vi "Periodic Tasks.vi"(8 "error in":errorcluster) -> ()   [LabVIEW 2020]
doc: "This VI runs in parallel to other tasks. It can contain as many user-defined periodic loops as you need. These can carry out PID or other sorts of timed response."
uses:
  <vilib>/Rock Robotics/WPI/ThirdParty/Phoenix-LabVIEW/Motor Controller/Controls/CTRE_Phoenix_MotorControl_ControlMode.ctl
  <vilib>/Analysis/coordinate.llb/Angle Range (Degree).ctl
  <vilib>/Analysis/coordinate.llb/Angle Units.ctl
  <vilib>/Analysis/coordinate.llb/Wrap Angle (scalar).vi
  globals.vi
  <vilib>/Rock Robotics/WPI/ThirdParty/Phoenix-LabVIEW/Pigeon IMU/CTRE_PigeonIMU_GetYPR.vi
  <vilib>/Rock Robotics/WPI/ThirdParty/Phoenix-LabVIEW/CANCoder/Get/CTRE_Phoenix_CANcoder_GetSensorData.vi
  <vilib>/Rock Robotics/WPI/ThirdParty/Phoenix-LabVIEW/CANCoder/Set/CTRE_Phoenix_CANcoder_SetPositionToAbsolute.vi
  <vilib>/Rock Robotics/WPI/ThirdParty/Phoenix-LabVIEW/Motor Controller/Get/CTRE_Phoenix_MotorController_GetSelectedSensorData.vi
  TitanLib/Lib/TitanLib.lvlib
  <vilib>/Analysis/NI_AAL_Angle.lvlib
panel:
  out "Pose Estimation (in) 3":cluster{"Pose[0]":dbl, "Pose[1]":dbl}[](graph)
  in  "wheel offset":dbl
  in  "Reset Odometry?":bool
  in  "Reset Encoders?":bool
  out "Encoders":dbl[](array[numeric])
  in  "Zero Pigeon?":bool
  out "Pose Estimation (in) 2":T1(graph)
  out "Pose Estimation (in)":cluster{"X":dbl, "Y":dbl}[](graph)
  in  "Drive Speed Multiplier":dbl=1.0
  in  "Enable Drive Motors?":bool=TRUE
  in  "Acceleration":i32=8192
  in  "Cruise Velocity":i32=20000
  in  "I":dbl
  in  "D":dbl=50.0
  in  "P":dbl=1.0
  in  "Set PIDF":bool
  out "Loop Time (ms)":u32(graph)
  # "Pos"
  # "Abs"
  # "Pos"
  # "Abs"
  # "Pos"
  # "Abs"
  # "Pos"
  # "Abs"
  # "30ft x 30ft"
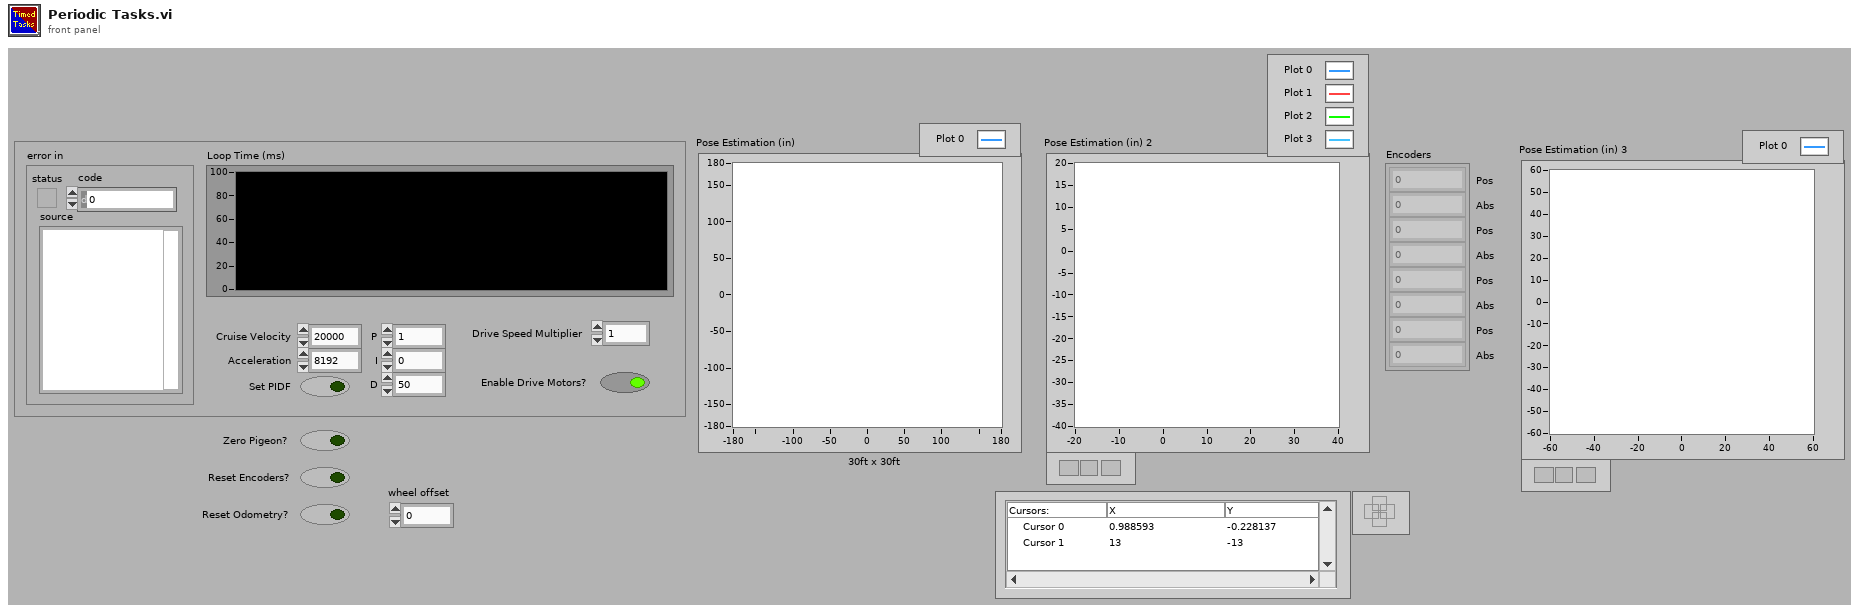
[diagram p1: front panel]
types:
  T1 = cluster{"output array":dbl[], "output array":dbl[]}[]
  T2 = typedef "WPI_MotorControlDeviceRef.ctl" = cluster{"DeviceStatus":errorcluster, "Type":T3, "PWM":cluster{"PWM Channel":T4, "DeadBand":T5}, "CAN":cluster{"Device Number":u8, "SetOutput VI Ref":variant, "GetOutput VI Ref":variant, "Enable VI Ref":variant, "Disable VI Ref":variant, "Data":variant}, "Invert":bool, "DIO PWM":cluster{"PWM \"Enable\" Channel":T4, "DIOChannel":T6, "PWM Rate":dbl}}
  T3 = typedef "WPI_MotorControlType.ctl" = enum16{"PWM", "CAN", "DIO PWM"}
  T4 = typedef "FPGA_DIOPWMChannel.ctl" = enum8{"PWM 0", "PWM 1", "PWM 2", "PWM 3", "PWM 4", "PWM 5", "PWM 6", "PWM 7", "PWM 8", "PWM 9", "PWM MXP 0", "PWM MXP 1", "PWM MXP 2", "PWM MXP 3", "PWM MXP 4", "PWM MXP 5", "PWM MXP 6", "PWM MXP 7", "PWM MXP 8", "PWM MXP 9", "Invalid"}
  T5 = typedef "WPI_PWMDeadband.ctl" = cluster{"Name":string, "maxPositivePwm":i32, "minPositivePwm":i32, "centerPwm":i32, "maxNegativePwm":i32, "minNegativePwm":i32, "angularRange":u16}
  T6 = typedef "FPGA_DIOChannel.ctl" = enum8{"DIO 0", "DIO 1", "DIO 2", "DIO 3", "DIO 4", "DIO 5", "DIO 6", "DIO 7", "DIO 8", "DIO 9", "DIO MXP 0", "DIO MXP 1", "DIO MXP 2", "DIO MXP 3", "DIO MXP 4", "DIO MXP 5", "DIO MXP 6", "DIO MXP 7", "DIO MXP 8", "DIO MXP 9", "DIO MXP 10", "DIO MXP 11", "DIO MXP 12", "DIO MXP 13", "DIO MXP 14", "DIO MXP 15", "SPI Port CS1", "SPI Port CS2", "SPI Port CS3", "SPI Port MISO", "SPI Port MOSI", "Invalid"}
  T7 = typedef "CTRE_Phoenix_CANcoder_DeviceRef.ctl" = cluster{"DeviceStatus":errorcluster, "Device Number":u8, "Handle":u64, "UsageFrame":u32, "Library Path":path}
  T8 = typedef "CTRE_PigeonIMU_DeviceRef.ctl" = cluster{"DeviceStatus":errorcluster, "Device Number":u8, "Type":T9, "Device ID":u32, "Handle":u64, "UsageFrame":u32, "Library Path":path}
  T9 = typedef "CTRE_PigeonIMU_ConnectionType.ctl" = u32
  T10 = typedef "NI_AAL_Angle.lvlib/Angle Units.ctl" = i32
  T11 = typedef "NI_AAL_Angle.lvlib/Angle Range (Degree).ctl" = u16
  T12 = typedef "CTRE_Phoenix_MotorControl_ControlMode.ctl" = u16
  T13 = cluster{"output array":dbl[], "output array":dbl[]}
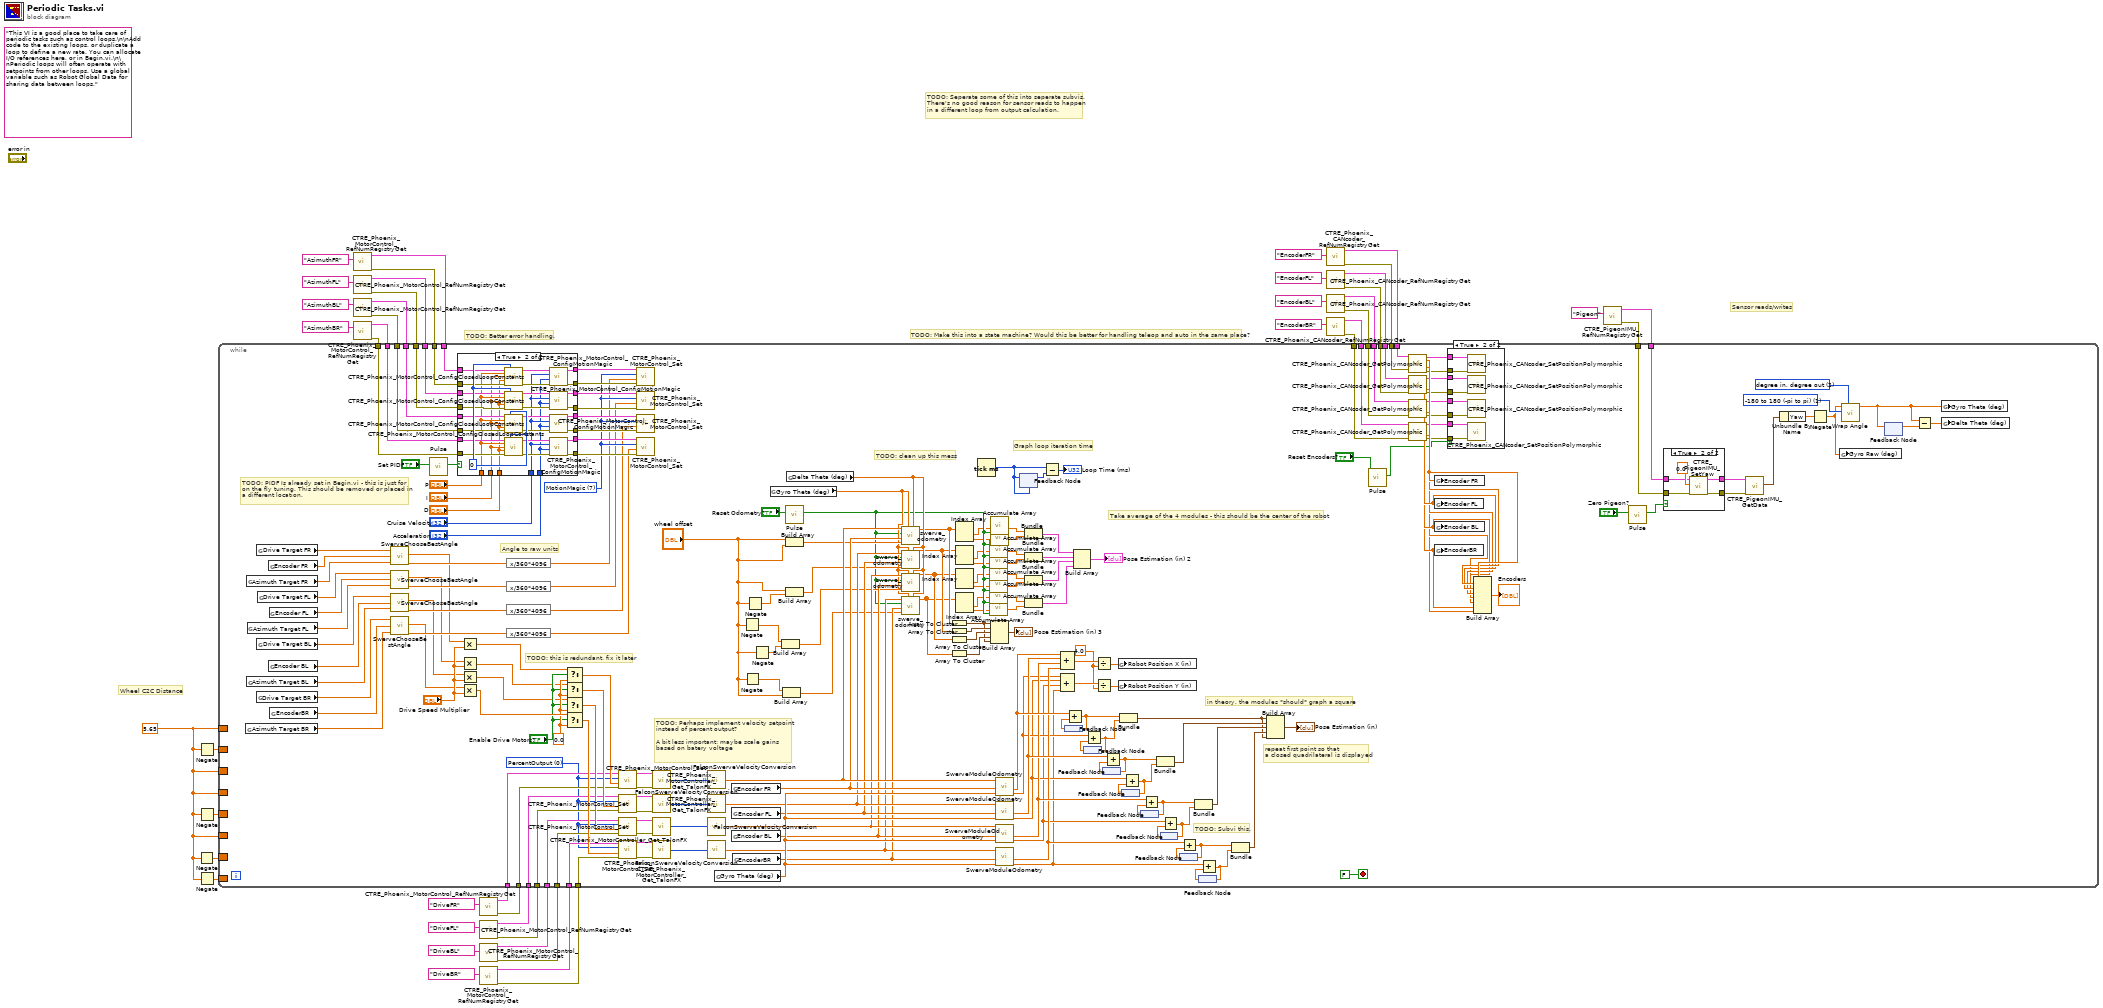
[diagram p0: block diagram]
diagram:
  w1 = 5.65
  (unwired) "This VI is a good place to take care of periodic tasks such as control loops.\n\nAdd code to the existing loops, or duplicate a loop to define a new rate. You can allocate I/O references here, or in Begin.vi.\n\nPeriodic loops will often operate with setpoints from other loops. Use a global variable such as Robot Global Data for sharing data between loops."
  # "Sensor reads/writes"
  # "TODO: Better error handling."
  # "TODO: Make this into a state machine? Would this be better for handling teleop and auto in the same place?"
  # "TODO: Seperate some of this into seperate subvis.\nThere's no good reason for sensor reads to happen\nin a different loop from output calculation."
  # "Wheel C2C Distance"
  n1 = Negate(x=w1) -> (-x=w17:dbl)
  n2 = Negate(x=w1) -> (-x=w18:dbl)
  n3 = Negate(x=w1) -> (-x=w20:dbl)
  n4 = Negate(x=w1) -> (-x=w19:dbl)
  n5 = call <vilib>:"CTRE_Phoenix_MotorControl_RefNumRegistryGet.vi"("refnum name"="AzimuthFR") -> ("error out"=w38:errorcluster, "PhoenixMotorControlDevRef"=w37:T2)  [unwired: 9 in]
  n6 = call <vilib>:"CTRE_Phoenix_MotorControl_RefNumRegistryGet.vi"("refnum name"="AzimuthFL") -> ("error out"=w40:errorcluster, "PhoenixMotorControlDevRef"=w39:T2)  [unwired: 9 in]
  n7 = call <vilib>:"CTRE_Phoenix_MotorControl_RefNumRegistryGet.vi"("refnum name"="AzimuthBL") -> ("error out"=w42:errorcluster, "PhoenixMotorControlDevRef"=w41:T2)  [unwired: 9 in]
  n8 = call <vilib>:"CTRE_Phoenix_MotorControl_RefNumRegistryGet.vi"("refnum name"="AzimuthBR") -> ("error out"=w44:errorcluster, "PhoenixMotorControlDevRef"=w43:T2)  [unwired: 9 in]
  n9 = call <vilib>:"CTRE_Phoenix_MotorControl_RefNumRegistryGet.vi"("refnum name"="DriveFR") -> ("error out"=w26:errorcluster, "PhoenixMotorControlDevRef"=w25:T2)  [unwired: 9 in]
  n10 = call <vilib>:"CTRE_Phoenix_MotorControl_RefNumRegistryGet.vi"("refnum name"="DriveFL") -> ("error out"=w28:errorcluster, "PhoenixMotorControlDevRef"=w27:T2)  [unwired: 9 in]
  n11 = call <vilib>:"CTRE_Phoenix_MotorControl_RefNumRegistryGet.vi"("refnum name"="DriveBL") -> ("error out"=w30:errorcluster, "PhoenixMotorControlDevRef"=w29:T2)  [unwired: 9 in]
  n12 = call <vilib>:"CTRE_Phoenix_MotorControl_RefNumRegistryGet.vi"("refnum name"="DriveBR") -> ("error out"=w32:errorcluster, "PhoenixMotorControlDevRef"=w31:T2)  [unwired: 9 in]
  n13 = call <vilib>:"CTRE_Phoenix_CANcoder_RefNumRegistryGet.vi"("refnum name"="EncoderFR") -> ("error out"=w6:errorcluster, "CTRE_CANcoder_DeviceRef"=w5:T7)  [unwired: 9 in]
  n14 = call <vilib>:"CTRE_Phoenix_CANcoder_RefNumRegistryGet.vi"("refnum name"="EncoderFL") -> ("error out"=w12:errorcluster, "CTRE_CANcoder_DeviceRef"=w11:T7)  [unwired: 9 in]
  n15 = call <vilib>:"CTRE_Phoenix_CANcoder_RefNumRegistryGet.vi"("refnum name"="EncoderBL") -> ("error out"=w8:errorcluster, "CTRE_CANcoder_DeviceRef"=w7:T7)  [unwired: 9 in]
  n16 = call <vilib>:"CTRE_Phoenix_CANcoder_RefNumRegistryGet.vi"("refnum name"="EncoderBR") -> ("error out"=w10:errorcluster, "CTRE_CANcoder_DeviceRef"=w9:T7)  [unwired: 9 in]
  n17 = call <vilib>:"CTRE_PigeonIMU_RefNumRegistryGet.vi"("refnum name"="Pigeon") -> ("error out"=w3:errorcluster, "PigeonIMUDevRef"=w2:T8)  [unwired: 9 in]
  n18 = while {
    tunnel: w44 -> [w210]
    tunnel: w43 -> [w209]
    tunnel: w42 -> [w208]
    tunnel: w41 -> [w207]
    tunnel: w40 -> [w206]
    tunnel: w39 -> [w205]
    tunnel: w38 -> [w204]
    tunnel: w37 -> [w203]
    tunnel: w32 -> [w202]
    tunnel: w31 -> [w201]
    tunnel: w30 -> [w200]
    tunnel: w29 -> [w199]
    tunnel: w28 -> [w198]
    tunnel: w27 -> [w197]
    tunnel: w26 -> [w196]
    tunnel: w25 -> [w195]
    border: w1 -> [_]
    border: w18 -> [_]
    border: w1 -> [_]
    border: w1 -> [_]
    border: w20 -> [_]
    border: w1 -> [_]
    border: w17 -> [_]
    border: w19 -> [_]
    tunnel: w12 -> [w150]
    tunnel: w11 -> [w149]
    tunnel: w10 -> [w148]
    tunnel: w9 -> [w147]
    tunnel: w8 -> [w146]
    tunnel: w7 -> [w145]
    tunnel: w6 -> [w144]
    tunnel: w5 -> [w143]
    tunnel: w3 -> [w142]
    tunnel: w2 -> [w141]
    stop <- FALSE stop-if-true
    w48 = 4.0 ("y")
    w157 = T10 2 items=["radian in, radian out", "radian in, degree out", "degree in, degree out", "degree in, radian out"] ("angle units")
    w156 = T11 1 items=["none", "-180 to 180 (-pi to pi)", "0 to 360 (0 to 2pi)"] ("angle range")
    w193 = T12 0 items=["PercentOutput"=0, "Position"=1, "Velocity"=2, "Current"=3, "Follower"=5, "MotionProfile"=6, "MotionMagic"=7, "MotionProfileArc"=10, "Disabled"=15] ("Control Mode")
    w194 = 0.0 ("f")
    w245 = T12 7 items=["PercentOutput"=0, "Position"=1, "Velocity"=2, "Current"=3, "Follower"=5, "MotionProfile"=6, "MotionMagic"=7, "MotionProfileArc"=10, "Disabled"=15] ("Control Mode")
    # "TODO: Subvi this."
    # "repeat first point so that\na closed quadrilateral is displayed"
    # "in theory, the modules *should* graph a square"
    # "Take average of the 4 modules - this should be the center of the robot"
    # "TODO: clean up this mess"
    # "TODO: Perhaps implement velocity setpoint\ninstead of percent output?\n\nA bit less important: maybe scale gains\nbased on batery voltage"
    # "TODO: this is redundant. fix it later"
    # "Graph loop iteration time"
    # "Angle to raw units"
    # "TODO: PIDF Is already set in Begin.vi - this is just for\non the fly tuning. This should be removed or placed in\na different location."
    n19 = global read "globals.vi" "Azimuth Target BR"() -> (w213:dbl)
    n20 = global read "globals.vi" "Azimuth Target FR"() -> (w219:dbl)
    n21 = global read "globals.vi" "Azimuth Target BL"() -> (w215:dbl)
    n22 = global read "globals.vi" "Azimuth Target FL"() -> (w217:dbl)
    n23 = global read "globals.vi" "Drive Target BR"() -> (w214:dbl)
    n24 = global read "globals.vi" "Drive Target FR"() -> (w181:dbl)
    n25 = global read "globals.vi" "Drive Target BL"() -> (w216:dbl)
    n26 = global read "globals.vi" "Drive Target FL"() -> (w218:dbl)
    n27 = global read "globals.vi" "Encoder FR"() -> (w180:dbl)
    n28 = global read "globals.vi" "Encoder BL"() -> (w178:dbl)
    n29 = global read "globals.vi" "Encoder FL"() -> (w179:dbl)
    n30 = global read "globals.vi" "EncoderBR"() -> (w177:dbl)
    n31 = call "SwerveChooseBestAngle.vi"("Target Angle"=w219, "Current Angle"=w180, "Power In"=w181) -> ("Setpoint Angle"=w239:dbl, "Power Out"=w228:dbl)  [unwired: 4 in]
    n32 = call "SwerveChooseBestAngle.vi"("Target Angle"=w217, "Current Angle"=w179, "Power In"=w218) -> ("Setpoint Angle"=w238:dbl, "Power Out"=w227:dbl)  [unwired: 4 in]
    n33 = call "SwerveChooseBestAngle.vi"("Target Angle"=w215, "Current Angle"=w178, "Power In"=w216) -> ("Setpoint Angle"=w237:dbl, "Power Out"=w226:dbl)  [unwired: 4 in]
    n34 = call "SwerveChooseBestAngle.vi"("Target Angle"=w213, "Current Angle"=w177, "Power In"=w214) -> ("Setpoint Angle"=w236:dbl, "Power Out"=w225:dbl)  [unwired: 4 in]
    n35 = call "Pulse.vi"("Input"="Set PIDF") -> ("Output"=w243:bool)  [unwired: 10 in]
    n36 = case shown="True" w243 {
      tunnel: [w277 w285] -> w253
      tunnel: [w278 w286] -> w252
      tunnel: [w276 w284] -> w251
      tunnel: [w275 w283] -> w250
      tunnel: [w273 w281] -> w249
      tunnel: [w274 w282] -> w248
      tunnel: [w272 w280] -> w247
      tunnel: [w271 w279] -> w246
      tunnel: w203 -> [w278 w307]
      tunnel: w204 -> [w277 w306]
      tunnel: w205 -> [w276 w305]
      tunnel: w206 -> [w275 w304]
      tunnel: w207 -> [w274 w303]
      tunnel: w208 -> [w273 w302]
      tunnel: w209 -> [w272 w301]
      tunnel: w210 -> [w271 w300]
      tunnel: "P" -> [_ w299]
      tunnel: "I" -> [_ w298]
      tunnel: "D" -> [_ w297]
      tunnel: "Cruise Velocity" -> [_ w288]
      tunnel: "Acceleration" -> [_ w287]
      frame False {
      }
      frame True {
        w308 = 0 ("slotIdx")
        n37 = call <vilib>:"CTRE_Phoenix_MotorControl_ConfigClosedLoopConstants.vi"("PhoenixMotorControlDevRef"=w307, "slotIdx"=w308, "P"=w299, "I"=w298, "D"=w297, "error in (no error)"=w306) -> ("PhoenixMotorControlDevRef"=w295:T2, "error out"=w296:errorcluster)  [unwired: 8 in]
        n38 = call <vilib>:"CTRE_Phoenix_MotorControl_ConfigClosedLoopConstants.vi"("PhoenixMotorControlDevRef"=w305, "slotIdx"=w308, "P"=w299, "I"=w298, "D"=w297, "error in (no error)"=w304) -> ("PhoenixMotorControlDevRef"=w293:T2, "error out"=w294:errorcluster)  [unwired: 8 in]
        n39 = call <vilib>:"CTRE_Phoenix_MotorControl_ConfigClosedLoopConstants.vi"("PhoenixMotorControlDevRef"=w303, "slotIdx"=w308, "P"=w299, "I"=w298, "D"=w297, "error in (no error)"=w302) -> ("PhoenixMotorControlDevRef"=w291:T2, "error out"=w292:errorcluster)  [unwired: 8 in]
        n40 = call <vilib>:"CTRE_Phoenix_MotorControl_ConfigClosedLoopConstants.vi"("PhoenixMotorControlDevRef"=w301, "slotIdx"=w308, "P"=w299, "I"=w298, "D"=w297, "error in (no error)"=w300) -> ("PhoenixMotorControlDevRef"=w289:T2, "error out"=w290:errorcluster)  [unwired: 8 in]
        n41 = call <vilib>:"CTRE_Phoenix_MotorControl_ConfigMotionMagic.vi"("error in (no error)"=w296, "Acceleration"=w287, "Cruise Velocity"=w288, "PhoenixMotorControlDevRef"=w295) -> ("error out"=w285:errorcluster, "PhoenixMotorControlDevRef"=w286:T2)  [unwired: 6 in]
        n42 = call <vilib>:"CTRE_Phoenix_MotorControl_ConfigMotionMagic.vi"("error in (no error)"=w294, "Acceleration"=w287, "Cruise Velocity"=w288, "PhoenixMotorControlDevRef"=w293) -> ("error out"=w283:errorcluster, "PhoenixMotorControlDevRef"=w284:T2)  [unwired: 6 in]
        n43 = call <vilib>:"CTRE_Phoenix_MotorControl_ConfigMotionMagic.vi"("error in (no error)"=w292, "Acceleration"=w287, "Cruise Velocity"=w288, "PhoenixMotorControlDevRef"=w291) -> ("error out"=w281:errorcluster, "PhoenixMotorControlDevRef"=w282:T2)  [unwired: 6 in]
        n44 = call <vilib>:"CTRE_Phoenix_MotorControl_ConfigMotionMagic.vi"("error in (no error)"=w290, "Acceleration"=w287, "Cruise Velocity"=w288, "PhoenixMotorControlDevRef"=w289) -> ("error out"=w279:errorcluster, "PhoenixMotorControlDevRef"=w280:T2)  [unwired: 6 in]
      }
    }
    n45 = Multiply(x=w228, y="Drive Speed Multiplier") -> (x*y=w211:dbl)
    n46 = Multiply(x=w227, y="Drive Speed Multiplier") -> (x*y=w129:dbl)
    n47 = Multiply(x=w226, y="Drive Speed Multiplier") -> (x*y=w128:dbl)
    n48 = Multiply(x=w225, y="Drive Speed Multiplier") -> (x*y=w224:dbl)
    n49 = expression code="x/360*4096"(w239) -> (w233:dbl)
    n50 = expression code="x/360*4096"(w238) -> (w232:dbl)
    n51 = expression code="x/360*4096"(w237) -> (w231:dbl)
    n52 = expression code="x/360*4096"(w236) -> (w230:dbl)
    n53 = Select(t=w211, s="Enable Drive Motors?", f=w194) -> (s? t:f=w220:dbl)
    n54 = Select(t=w129, s="Enable Drive Motors?", f=w194) -> (s? t:f=w221:dbl)
    n55 = Select(t=w128, s="Enable Drive Motors?", f=w194) -> (s? t:f=w222:dbl)
    n56 = Select(t=w224, s="Enable Drive Motors?", f=w194) -> (s? t:f=w223:dbl)
    n57 = call <vilib>:"CTRE_Phoenix_MotorControl_Set.vi"("error in (no error)"=w196, "Output"=w220, "Control Mode"=w193, "PhoenixMotorControlDevRef"=w195) -> ("error out"=w190:errorcluster, "PhoenixMotorControlDevRef"=w191:T2)  [unwired: 6 in]
    n58 = call <vilib>:"CTRE_Phoenix_MotorControl_Set.vi"("error in (no error)"=w198, "Output"=w221, "Control Mode"=w193, "PhoenixMotorControlDevRef"=w197) -> ("error out"=w188:errorcluster, "PhoenixMotorControlDevRef"=w189:T2)  [unwired: 6 in]
    n59 = call <vilib>:"CTRE_Phoenix_MotorControl_Set.vi"("error in (no error)"=w200, "Output"=w222, "Control Mode"=w193, "PhoenixMotorControlDevRef"=w199) -> ("error out"=w186:errorcluster, "PhoenixMotorControlDevRef"=w187:T2)  [unwired: 6 in]
    n60 = call <vilib>:"CTRE_Phoenix_MotorControl_Set.vi"("error in (no error)"=w202, "Output"=w223, "Control Mode"=w193, "PhoenixMotorControlDevRef"=w201) -> ("error out"=w184:errorcluster, "PhoenixMotorControlDevRef"=w185:T2)  [unwired: 6 in]
    n61 = call <vilib>:"CTRE_Phoenix_MotorControl_Set.vi"("error in (no error)"=w253, "Output"=w233, "Control Mode"=w245, "PhoenixMotorControlDevRef"=w252) -> ()  [unwired: 6 in, 2 out]
    n62 = call <vilib>:"CTRE_Phoenix_MotorControl_Set.vi"("error in (no error)"=w250, "Output"=w232, "Control Mode"=w245, "PhoenixMotorControlDevRef"=w251) -> ()  [unwired: 6 in, 2 out]
    n63 = call <vilib>:"CTRE_Phoenix_MotorControl_Set.vi"("error in (no error)"=w249, "Output"=w231, "Control Mode"=w245, "PhoenixMotorControlDevRef"=w248) -> ()  [unwired: 6 in, 2 out]
    n64 = call <vilib>:"CTRE_Phoenix_MotorControl_Set.vi"("error in (no error)"=w246, "Output"=w230, "Control Mode"=w245, "PhoenixMotorControlDevRef"=w247) -> ()  [unwired: 6 in, 2 out]
    n65 = call-poly <vilib>:"CTRE_Phoenix_MotorController_Get_TalonFX.vi"("PhoenixMotorControlDevRef"=w191, "error in"=w190) -> ("Velocity (Raw Sensor Units per 100 ms)"=w182:i32)  [unwired: 10 in, 3 out]
    n66 = call-poly <vilib>:"CTRE_Phoenix_MotorController_Get_TalonFX.vi"("PhoenixMotorControlDevRef"=w189, "error in"=w188) -> ("Velocity (Raw Sensor Units per 100 ms)"=w139:i32)  [unwired: 10 in, 3 out]
    n67 = call-poly <vilib>:"CTRE_Phoenix_MotorController_Get_TalonFX.vi"("PhoenixMotorControlDevRef"=w187, "error in"=w186) -> ("Velocity (Raw Sensor Units per 100 ms)"=w138:i32)  [unwired: 10 in, 3 out]
    n68 = call-poly <vilib>:"CTRE_Phoenix_MotorController_Get_TalonFX.vi"("PhoenixMotorControlDevRef"=w185, "error in"=w184) -> ("Velocity (Raw Sensor Units per 100 ms)"=w183:i32)  [unwired: 10 in, 3 out]
    n69 = call "FalconSwerveVelocityConversion.vi"("Velocity (Raw Sensor Units per 100 ms)"=w182) -> ("Velocity (ft/s)"=w175:dbl)
    n70 = call "FalconSwerveVelocityConversion.vi"("Velocity (Raw Sensor Units per 100 ms)"=w139) -> ("Velocity (ft/s)"=w173:dbl)
    n71 = call "FalconSwerveVelocityConversion.vi"("Velocity (Raw Sensor Units per 100 ms)"=w138) -> ("Velocity (ft/s)"=w171:dbl)
    n72 = call "FalconSwerveVelocityConversion.vi"("Velocity (Raw Sensor Units per 100 ms)"=w183) -> ("Velocity (ft/s)"=w169:dbl)
    n73 = global read "globals.vi" "Gyro Theta (deg)"() -> (w176:dbl)
    n74 = global read "globals.vi" "Encoder FR"() -> (w174:dbl)
    n75 = global read "globals.vi" "Encoder BL"() -> (w170:dbl)
    n76 = global read "globals.vi" "Encoder FL"() -> (w172:dbl)
    n77 = global read "globals.vi" "EncoderBR"() -> (w168:dbl)
    n78 = Negate(x="wheel offset") -> (-x=w167:dbl)
    n79 = Negate(x="wheel offset") -> (-x=w140:dbl)
    n80 = Negate(x="wheel offset") -> (-x=w114:dbl)
    n81 = Negate(x="wheel offset") -> (-x=w113:dbl)
    n82 = global read "globals.vi" "Gyro Theta (deg)"() -> (w116:dbl)
    n83 = Build Array(w167, w113) -> (w164:dbl[])
    n84 = Build Array(w140, "wheel offset") -> (w163:dbl[])
    n85 = call "Pulse.vi"("Input"="Reset Odometry?") -> ("Output"=w112:bool)  [unwired: 10 in]
    n86 = Build Array("wheel offset", "wheel offset") -> (w166:dbl[])
    n87 = Build Array("wheel offset", w114) -> (w165:dbl[])
    n88 = global read "globals.vi" "Delta Theta (deg)"() -> (w115:dbl)
    n89 = call "swerve_odometry.vi"("Delta Theta (deg)"=w115, "Gyro Theta (deg)"=w116, "wheel pos"=w166, "Wheel Azimuth (deg)"=w174, "Reset?"=w112, "Wheel Velocity (ft/s)"=w175) -> ("Pose"=w110:dbl[])  [unwired: 5 in]
    n90 = call "swerve_odometry.vi"("Delta Theta (deg)"=w115, "Gyro Theta (deg)"=w116, "wheel pos"=w165, "Wheel Azimuth (deg)"=w172, "Reset?"=w112, "Wheel Velocity (ft/s)"=w173) -> ("Pose"=w109:dbl[])  [unwired: 5 in]
    n91 = call "swerve_odometry.vi"("Delta Theta (deg)"=w115, "Gyro Theta (deg)"=w116, "wheel pos"=w164, "Wheel Azimuth (deg)"=w170, "Reset?"=w112, "Wheel Velocity (ft/s)"=w171) -> ("Pose"=w108:dbl[])  [unwired: 5 in]
    n92 = call "swerve_odometry.vi"("Delta Theta (deg)"=w115, "Gyro Theta (deg)"=w116, "wheel pos"=w163, "Wheel Azimuth (deg)"=w168, "Reset?"=w112, "Wheel Velocity (ft/s)"=w169) -> ("Pose"=w107:dbl[])  [unwired: 5 in]
    n93 = Array To Cluster(array=w110) -> (cluster=w103:cluster{"Pose[0]":dbl, "Pose[1]":dbl})
    n94 = Array To Cluster(array=w109) -> (cluster=w106:cluster{"Pose[0]":dbl, "Pose[1]":dbl})
    n95 = Array To Cluster(array=w108) -> (cluster=w105:cluster{"Pose[0]":dbl, "Pose[1]":dbl})
    n96 = Array To Cluster(array=w107) -> (cluster=w104:cluster{"Pose[0]":dbl, "Pose[1]":dbl})
    n97 = Index Array(array=w109) -> (element #1=w95:dbl, element #2=w96:dbl)  [unwired: 2 in]
    n98 = Index Array(array=w108) -> (element #1=w94:dbl, element #2=w93:dbl)  [unwired: 2 in]
    n99 = Index Array(array=w107) -> (element #1=w91:dbl, element #2=w92:dbl)  [unwired: 2 in]
    n100 = Index Array(array=w110) -> (element #1=w100:dbl, element #2=w99:dbl)  [unwired: 2 in]
    n101 = Tick Count (ms)() -> (millisecond timer value=w101:u32)
    n102 = call "Accumulate Array.vi"("Reset?"=w112, "value"=w95) -> ("output array"=w85:dbl[])  [unwired: 9 in]
    n103 = call "Accumulate Array.vi"("Reset?"=w112, "value"=w96) -> ("output array"=w86:dbl[])  [unwired: 9 in]
    n104 = call "Accumulate Array.vi"("Reset?"=w112, "value"=w94) -> ("output array"=w87:dbl[])  [unwired: 9 in]
    n105 = call "Accumulate Array.vi"("Reset?"=w112, "value"=w93) -> ("output array"=w88:dbl[])  [unwired: 9 in]
    n106 = call "Accumulate Array.vi"("Reset?"=w112, "value"=w91) -> ("output array"=w90:dbl[])  [unwired: 9 in]
    n107 = call "Accumulate Array.vi"("Reset?"=w112, "value"=w92) -> ("output array"=w89:dbl[])  [unwired: 9 in]
    n108 = call "Accumulate Array.vi"("Reset?"=w112, "value"=w100) -> ("output array"=w98:dbl[])  [unwired: 9 in]
    n109 = call "Accumulate Array.vi"("Reset?"=w112, "value"=w99) -> ("output array"=w97:dbl[])  [unwired: 9 in]
    n110 = Build Array(w103, w106, w105, w104, w103) -> (→"Pose Estimation (in) 3":cluster{"Pose[0]":dbl, "Pose[1]":dbl}[])
    n111 = call "SwerveModuleOdometry.vi"("Robot Heading(deg)"=w176, "Wheel Azimuth (deg)"=w174, "Velocity (ft/s)"=w175) -> ("Delta Y (in)"=w54:dbl, "Delta X (in)"=w58:dbl)  [unwired: 3 in, 2 out]
    n112 = call "SwerveModuleOdometry.vi"("Robot Heading(deg)"=w176, "Wheel Azimuth (deg)"=w172, "Velocity (ft/s)"=w173) -> ("Delta Y (in)"=w53:dbl, "Delta X (in)"=w57:dbl)  [unwired: 3 in, 2 out]
    n113 = call "SwerveModuleOdometry.vi"("Robot Heading(deg)"=w176, "Wheel Azimuth (deg)"=w170, "Velocity (ft/s)"=w171) -> ("Delta Y (in)"=w52:dbl, "Delta X (in)"=w56:dbl)  [unwired: 3 in, 2 out]
    n114 = call "SwerveModuleOdometry.vi"("Robot Heading(deg)"=w176, "Wheel Azimuth (deg)"=w168, "Velocity (ft/s)"=w169) -> ("Delta Y (in)"=w51:dbl, "Delta X (in)"=w55:dbl)  [unwired: 3 in, 2 out]
    n115 = feedback #1(w101) -> (w255:u32)
    n116 = feedback-in #1(w101) -> ()
    n117 = Bundle("output array"=w98, "output array"=w97) -> (w84:T13)  [unwired: 1 in]
    n118 = Bundle("output array"=w85, "output array"=w86) -> (w83:T13)  [unwired: 1 in]
    n119 = Bundle("output array"=w87, "output array"=w88) -> (w82:T13)  [unwired: 1 in]
    n120 = Bundle("output array"=w90, "output array"=w89) -> (w81:T13)  [unwired: 1 in]
    n121 = Subtract(x=w101, y=w255) -> (x-y=→"Loop Time (ms)":u32)
    n122 = Compound Arithmetic op=ADD(w58, w57, w56, w55) -> (w49:dbl)
    n123 = Compound Arithmetic op=ADD(w54, w53, w52, w51) -> (w50:dbl)
    n124 = feedback #2() -> (w79:dbl)
    n125 = Add(x=w58, y=w79) -> (x+y=w71:dbl)
    n126 = feedback-in #2(w71) -> ()
    n127 = Build Array(w84, w83, w82, w81) -> (→"Pose Estimation (in) 2":T1)
    n128 = feedback #3() -> (w78:dbl)
    n129 = Add(x=w54, y=w78) -> (x+y=w70:dbl)
    n130 = feedback-in #3(w70) -> ()
    n131 = Divide(x=w49, y=w48) -> (x/y=w47:dbl)
    n132 = Divide(x=w50, y=w48) -> (x/y=w46:dbl)
    n133 = feedback #4() -> (w76:dbl)
    n134 = Add(x=w57, y=w76) -> (x+y=w69:dbl)
    n135 = feedback-in #4(w69) -> ()
    n136 = global write "globals.vi" "Robot Position X (in)"(w47) -> ()
    n137 = global write "globals.vi" "Robot Position Y (in)"(w46) -> ()
    n138 = Bundle(w71, w70) -> (w59:cluster{dbl, dbl})  [unwired: 1 in]
    n139 = feedback #5() -> (w77:dbl)
    n140 = Add(x=w53, y=w77) -> (x+y=w68:dbl)
    n141 = feedback-in #5(w68) -> ()
    n142 = feedback #6() -> (w75:dbl)
    n143 = Add(x=w56, y=w75) -> (x+y=w67:dbl)
    n144 = feedback-in #6(w67) -> ()
    n145 = Bundle(w69, w68) -> (w61:cluster{dbl, dbl})  [unwired: 1 in]
    n146 = feedback #7() -> (w74:dbl)
    n147 = Add(x=w52, y=w74) -> (x+y=w66:dbl)
    n148 = feedback-in #7(w66) -> ()
    n149 = feedback #8() -> (w73:dbl)
    n150 = Add(x=w55, y=w73) -> (x+y=w65:dbl)
    n151 = feedback-in #8(w65) -> ()
    n152 = Bundle(w67, w66) -> (w62:cluster{dbl, dbl})  [unwired: 1 in]
    n153 = feedback #9() -> (w72:dbl)
    n154 = Add(x=w51, y=w72) -> (x+y=w64:dbl)
    n155 = feedback-in #9(w64) -> ()
    n156 = Bundle(w65, w64) -> (w63:cluster{dbl, dbl})  [unwired: 1 in]
    n157 = Build Array(w59, w61, w62, w63, w59) -> (→"Pose Estimation (in)":cluster{dbl, dbl}[])
    n158 = call "Pulse.vi"("Input"="Reset Encoders?") -> ("Output"=w118:bool)  [unwired: 10 in]
    n159 = call-poly <vilib>:"CTRE_Phoenix_CANcoder_GetPolymorphic.vi"("CTRE_CANcoder_DeviceRef"=w143, "error in"=w144) -> ("CTRE_CANcoder_DeviceRef"=w127:T7, "Position"=w137:dbl, "Absolute Position"=w136:dbl, "error out"=w126:errorcluster)  [unwired: 9 in, 1 out]
    n160 = call-poly <vilib>:"CTRE_Phoenix_CANcoder_GetPolymorphic.vi"("CTRE_CANcoder_DeviceRef"=w149, "error in"=w150) -> ("CTRE_CANcoder_DeviceRef"=w125:T7, "Position"=w135:dbl, "Absolute Position"=w134:dbl, "error out"=w124:errorcluster)  [unwired: 9 in, 1 out]
    n161 = call-poly <vilib>:"CTRE_Phoenix_CANcoder_GetPolymorphic.vi"("CTRE_CANcoder_DeviceRef"=w145, "error in"=w146) -> ("CTRE_CANcoder_DeviceRef"=w123:T7, "Position"=w133:dbl, "Absolute Position"=w132:dbl, "error out"=w122:errorcluster)  [unwired: 9 in, 1 out]
    n162 = call-poly <vilib>:"CTRE_Phoenix_CANcoder_GetPolymorphic.vi"("CTRE_CANcoder_DeviceRef"=w147, "error in"=w148) -> ("CTRE_CANcoder_DeviceRef"=w121:T7, "Position"=w131:dbl, "Absolute Position"=w130:dbl, "error out"=w120:errorcluster)  [unwired: 9 in, 1 out]
    n163 = global write "globals.vi" "Encoder FR"(w137) -> ()
    n164 = global write "globals.vi" "Encoder FL"(w135) -> ()
    n165 = global write "globals.vi" "Encoder BL"(w133) -> ()
    n166 = global write "globals.vi" "EncoderBR"(w131) -> ()
    n167 = case shown="True" w118 {
      tunnel: w127 -> [_ w263]
      tunnel: w126 -> [_ w262]
      tunnel: w125 -> [_ w261]
      tunnel: w124 -> [_ w260]
      tunnel: w123 -> [_ w259]
      tunnel: w122 -> [_ w258]
      tunnel: w121 -> [_ w257]
      tunnel: w120 -> [_ w256]
      frame False {
      }
      frame True {
        n168 = call-poly <vilib>:"CTRE_Phoenix_CANcoder_SetPositionPolymorphic.vi"("error in (no error)"=w262, "CTRE_CANcoder_DeviceRef"=w263) -> ()  [unwired: 8 in, 2 out]
        n169 = call-poly <vilib>:"CTRE_Phoenix_CANcoder_SetPositionPolymorphic.vi"("error in (no error)"=w260, "CTRE_CANcoder_DeviceRef"=w261) -> ()  [unwired: 8 in, 2 out]
        n170 = call-poly <vilib>:"CTRE_Phoenix_CANcoder_SetPositionPolymorphic.vi"("error in (no error)"=w258, "CTRE_CANcoder_DeviceRef"=w259) -> ()  [unwired: 8 in, 2 out]
        n171 = call-poly <vilib>:"CTRE_Phoenix_CANcoder_SetPositionPolymorphic.vi"("error in (no error)"=w256, "CTRE_CANcoder_DeviceRef"=w257) -> ()  [unwired: 8 in, 2 out]
      }
    }
    n172 = Build Array(w137, w136, w135, w134, w133, w132, w131, w130) -> (→"Encoders":dbl[])
    n173 = call "Pulse.vi"("Input"="Zero Pigeon?") -> ("Output"=w155:bool)  [unwired: 10 in]
    n174 = case shown="True" w155 {
      tunnel: w141 -> [w265 w269]
      tunnel: w142 -> [w264 w268]
      tunnel: [w265 w267] -> w160
      tunnel: [w264 w266] -> w161
      frame False {
      }
      frame True {
        n175 = call <vilib>:"CTRE_PigeonIMU_SetYaw.vi"("error in (no error)"=w268, "Value"=0.0, "PigeonIMUDevRef"=w269) -> ("error out"=w266:errorcluster, "PigeonIMUDevRef"=w267:T8)  [unwired: 7 in]
      }
    }
    n176 = call-poly <vilib>:"CTRE_PigeonIMU_GetData.vi"("error in (no error)"=w161, "PigeonIMUDevRef"=w160) -> ("Yaw Pitch Roll"=w162:cluster{"Yaw":dbl, "Pitch":dbl, "Roll":dbl})  [unwired: 7 in, 2 out]
    n177 = Unbundle By Name(w162) -> ("Yaw"=w158:dbl)
    n178 = Negate(x=w158) -> (-x=w154:dbl)
    n179 = global write "globals.vi" "Gyro Raw (deg)"(w154) -> ()
    n180 = call-poly <vilib>:"Wrap Angle.vi"("angle units"=w157, "angle range"=w156, "angle in"=w154) -> ("angle out"=w151:dbl)  [unwired: 7 in, 1 out]
    n181 = feedback #10() -> (w152:dbl)  [unwired: 1 in]
    n182 = feedback-in #10(w151) -> ()
    n183 = Subtract(x=w151, y=w152) -> (x-y=w153:dbl)
    n184 = global write "globals.vi" "Gyro Theta (deg)"(w151) -> ()
    n185 = global write "globals.vi" "Delta Theta (deg)"(w153) -> ()
  }
